vi "Create Exit Notifiers.vi"(8 "error in":errorcluster) -> (0 "error out":errorcluster, 3 "Notifiers":T1)   [LabVIEW 2015, in "PLC Notifiers.lvlib"]
uses:
  PLC Notifiers.lvlib
  PLC Notifiers.ctl
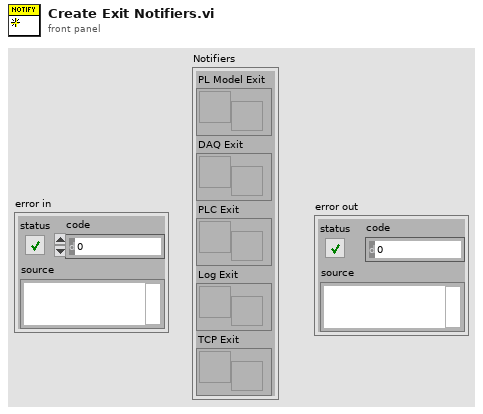
[diagram p1: front panel]
types:
  T1 = typedef "PLC Notifiers.lvlib/PLC Notifiers.ctl" = cluster{"PL Model Exit":refnum<notifier>, "DAQ Exit":refnum<notifier>, "PLC Exit":refnum<notifier>, "Log Exit":refnum<notifier>, "TCP Exit":refnum<notifier>}
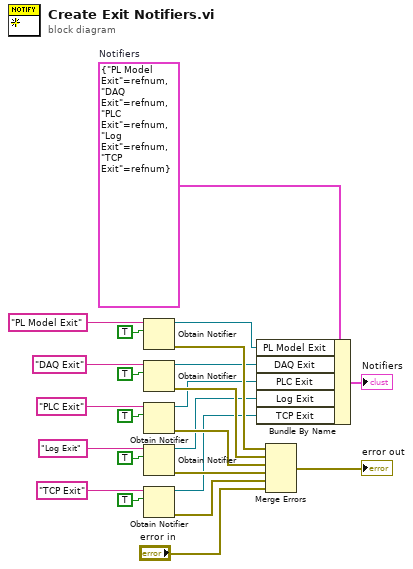
[diagram p0: block diagram]
diagram:
  w21 = T1 {"PL Model Exit"=refnum, "DAQ Exit"=refnum, "PLC Exit"=refnum, "Log Exit"=refnum, "TCP Exit"=refnum}  # Notifiers
  n1 = Obtain Notifier(name (unnamed)="PL Model Exit", notification data type=TRUE) -> (notifier out=w12:refnum<notifier>, error out=w23:errorcluster)  [unwired: 2 in, 1 out]
  n2 = Obtain Notifier(name (unnamed)="DAQ Exit", notification data type=TRUE) -> (notifier out=w11:refnum<notifier>, error out=w19:errorcluster)  [unwired: 2 in, 1 out]
  n3 = Obtain Notifier(name (unnamed)="PLC Exit", notification data type=TRUE) -> (notifier out=w10:refnum<notifier>, error out=w16:errorcluster)  [unwired: 2 in, 1 out]
  n4 = Obtain Notifier(name (unnamed)="Log Exit", notification data type=TRUE ("create if not found? (T)")) -> (notifier out=w8:refnum<notifier>, error out=w7:errorcluster)  [unwired: 2 in, 1 out]
  n5 = Obtain Notifier(name (unnamed)="TCP Exit", notification data type=TRUE ("create if not found? (T)")) -> (notifier out=w3:refnum<notifier>, error out=w2:errorcluster)  [unwired: 2 in, 1 out]
  n6 = Bundle By Name(cluster=w21, "PL Model Exit"=w12, "DAQ Exit"=w11, "PLC Exit"=w10, "Log Exit"=w8, "TCP Exit"=w3) -> (→"Notifiers":T1)
  n7 = Merge Errors(w23, w19, w16, w7, w2, "error in") -> (→"error out":errorcluster)
